vi "GET_PRESTATUS.vi"(10 "CODE_ID":string, 11 "PRODUCT_ID":string) -> (2 "字符串":string, 3 "OK?":bool)   [LabVIEW 2020]
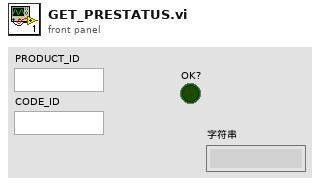
[diagram p1: front panel]
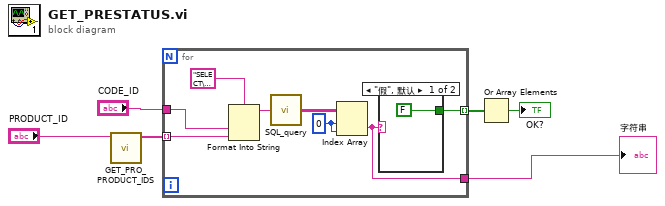
[diagram p0: block diagram]
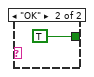
[diagram p2: hidden frame]
diagram:
  n1 = call "GET_PRO_PRODUCT_IDS.vi"("PRODUCT_ID"="PRODUCT_ID") -> ("前序工位"=w5:string[])  [unwired: 10 in]
  n2 = for {
    tunnel: w5 -> [w13] mode=indexing
    tunnel: "CODE_ID" -> [w12]
    tunnel: [w8] -> w3 mode=indexing
    tunnel: [w7] -> w1
    w9 = 0 ("索引 (行)")
    n3 = Format Into String(format string="SELECT\ndbo.Result.RESULT_VALUE\n\nFROM\ndbo.Result\nWHERE\ndbo.Result.CODE_ID = %s AND\ndbo.Result.DEVICE_ID = %s\n" ("格式字符串"), w12, w13) -> (resulting string=w11:string)  [unwired: 2 in, 1 out]
    n4 = call "SQL_query.vi"("SQL query"=w11) -> ("data"=w10:string[][])  [unwired: 3 in, 1 out]
    n5 = Index Array(array=w10, index (row)=w9, index (col)=w9) -> (element=w7:string)
    n6 = case shown="\"假\", 默认" w7 {
      tunnel: [FALSE TRUE] -> w8
      frame "假", Default {
      }
      frame "OK" {
      }
    }
  }
  "字符串" <- w1
  n7 = Or Array Elements(Boolean array=w3) -> (logical OR=→"OK?":bool)
